vi "ex_8.vi"() -> ()   [LabVIEW 2020]
panel:
  out "x+y":i32
  in  "String 2":string
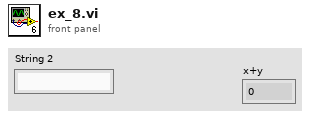
[diagram p1: front panel]
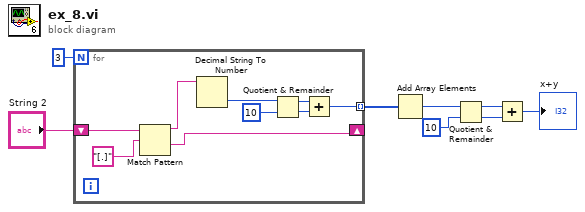
[diagram p0: block diagram]
diagram:
  n1 = for {
    N: 3 -> [_]
    shift-right: [w15] -> _
    shift-left: "String 2" -> [w17]
    tunnel: [w9] -> w6 mode=indexing
    n2 = Match Pattern(string=w17, regular expression="[.]") -> (before substring=w14:string, after substring=w15:string)  [unwired: 1 in, 2 out]
    n3 = Decimal String To Number(string=w14) -> (number=w13:i32)  [unwired: 2 in, 1 out]
    n4 = Quotient & Remainder(x=w13, y=10) -> (x-y*floor(x/y)=w11:i32, floor(x/y)=w10:i32)
    n5 = Add(x=w11, y=w10) -> (x+y=w9:i32)
  }
  n6 = Add Array Elements(numeric array=w6) -> (sum=w4:i32)
  n7 = Quotient & Remainder(x=w4, y=10) -> (x-y*floor(x/y)=w3:i32, floor(x/y)=w2:i32)
  n8 = Add(x=w3, y=w2) -> (x+y=→"x+y":i32)
